vi "Vision 차선 시프팅, 좌표변환.vi"(4 "Vision shift (m)":dbl, 5 "VIsion Lane":dbl[][](array[numeric])) -> (0 "theta":dbl[](array[numeric]), 1 "r":dbl[](array[numeric]), 2 "Vision":dbl[][](array[numeric]))   [LabVIEW 2016]
uses:
  <vilib>/imath/engines/lvmath2/RunTimeEngine/IndexRead/NIMS M($,S).vi
  <instcachedir>/0/NIMS M($,S)_3E5749BBB62E49528D4765A77F1F6D98.lvgen/NIMS M($,S)_3E5749BBB62E49528D4765A77F1F6D98_000.vi
  <vilib>/imathl/engines/lvmath/Functions/Error Handling/Create Error.vi
  <vilib>/imath/engines/lvmath2/RunTimeEngine/ArithmeticOperatorToken/NIMS_ArithmeticOperator_times.vi
  <instcachedir>/0/NIMS_ArithmeticOperator_times_953B34F74CAC448FB707D816A29CC5F0.lvgen/NIMS_ArithmeticOperator_times_953B34F74CAC448FB707D816A29CC5F0_000.vi
  <vilib>/imath/engines/lvmath2/RunTimeEngine/ArithmeticOperatorToken/NIMS_ArithmeticOperator_rightdiv.vi
  <instcachedir>/0/NIMS_ArithmeticOperator_rightdiv_0403F5D95ED04A4080FE3DA43A6A83B7.lvgen/NIMS_ArithmeticOperator_rightdiv_0403F5D95ED04A4080FE3DA43A6A83B7_000.vi
  <vilib>/imath/engines/lvmath2/RunTimeEngine/ErrorHandling/NIMS_Create Error From Enums.vi
  <vilib>/imath/engines/lvmath2/RunTimeEngine/ArithmeticOperatorToken/NIMS_ArithmeticOperator_plus.vi
  <instcachedir>/0/NIMS_ArithmeticOperator_plus_0120E0498A0F4B4B9BDCAC2554767A4E.lvgen/NIMS_ArithmeticOperator_plus_0120E0498A0F4B4B9BDCAC2554767A4E_004.vi
  <vilib>/imath/engines/lvmath2/RunTimeEngine/RowToken/NIMS_RowToken_CV_CV.vi
  <instcachedir>/0/NIMS_RowToken_CV_CV_5546A0B1CA2C4E49826F811B9C073FB0.lvgen/NIMS_RowToken_CV_CV_5546A0B1CA2C4E49826F811B9C073FB0_001.vi
  <vilib>/imath/engines/lvmath2/RunTimeEngine/NodeEndStatement/NIMS_NodeEndStatement_Output.vi
  <instcachedir>/0/NIMS_NodeEndStatement_Output_53EC0D466D134D7ABD903AC30B43404B.lvgen/NIMS_NodeEndStatement_Output_53EC0D466D134D7ABD903AC30B43404B_003.vi
  <instcachedir>/0/NIMS_NodeEndStatement_Output_53EC0D466D134D7ABD903AC30B43404B.lvgen/NIMS_NodeEndStatement_Output_53EC0D466D134D7ABD903AC30B43404B_000.vi
  <vilib>/imath/engines/lvmath2/RunTimeEngine/ErrorHandling/NIMS_Finalize Error.vi
panel:
  out "에러 출력":errorcluster
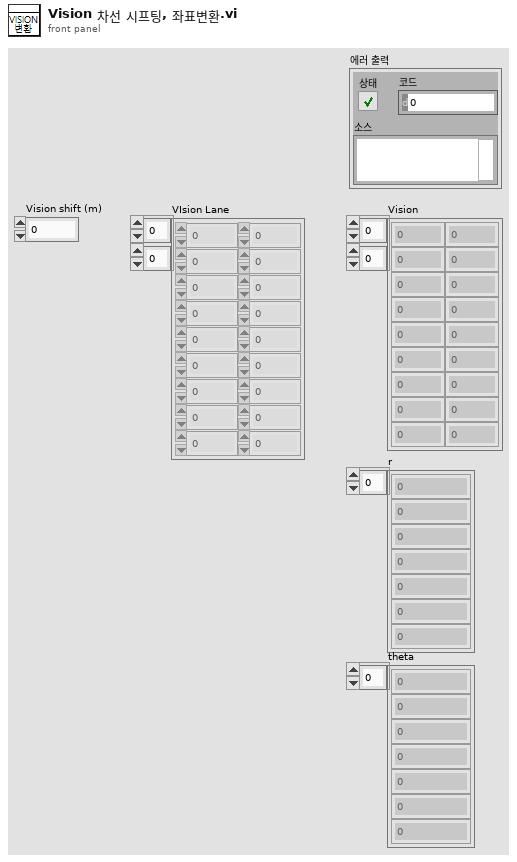
[diagram p1: front panel]
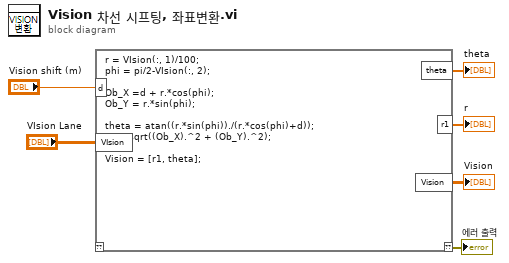
[diagram p0: block diagram]
diagram:
  n1 = mathscript code="r = VIsion(:, 1)/100;\nphi = pi/2-VIsion(:, 2);\n\nOb_X =d + r.*cos(phi);\nOb_Y = r.*sin(phi);\n\ntheta = atan((r.*sin(phi))./(r.*cos(phi)+d));\nr1 = sqrt((Ob_X).^2 + (Ob_Y).^2);\n\nVision = [r1, theta];"("d"="Vision shift (m)", "VIsion"="VIsion Lane") -> ("??"=→"에러 출력":errorcluster, "r1"=→"r":cdb[], "theta"=→"theta":cdb[], "Vision"=→"Vision":cdb[][])  [unwired: 1 in]
